vi "Cleanup Child.vi"(8 "error in (no error)":errorcluster, 11 "Install in":refnum<class "Install.lvclass">) -> (0 "error out":errorcluster, 3 "Install out":refnum<class "Install.lvclass">)   [LabVIEW 2020, in "Install.lvlib" / "Install.lvclass"]
uses:
  Install.lvclass
  build/ppl/neg-pkg.lvlibp/Action/Action.lvclass
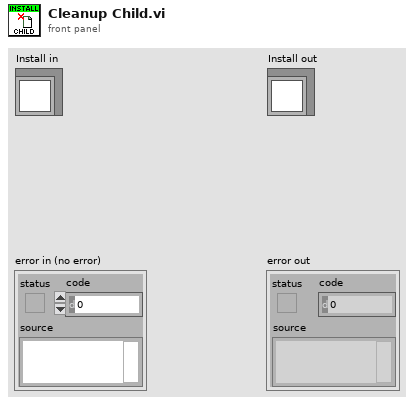
[diagram p1: front panel]
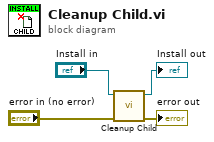
[diagram p0: block diagram]
diagram:
  n1 = call-parent "Cleanup Child.vi"("error in (no error)"="error in (no error)", "Action in"="Install in") -> ("error out"=→"error out":errorcluster, "Action out"=→"Install out":refnum<class "Install.lvclass">)  [unwired: 8 in]
